vi "UI exit.vi"(0 "ZenGage v3.0 UI in":T2, 1 "SM_Stop_Stop_UI":bool, 5 "Event Registration Refnum":refnum<event-registration>, 7 "User Events Cluster_UI":T1, 9 "This VI":refnum<vi>, 11 "error in (no error)":errorcluster, 12 "SlaveLoop_UI":refnum<user-event>) -> (4 "ZenGage v3.0 UI out":T2, 6 "Stop Actor Loop":bool, 15 "error out":errorcluster)   [LabVIEW 2019, in "ZenGage v3.0 UI.lvclass"]
uses:
  ZenGage v3.0 UI.lvclass
  Type Definitions/User Events UI/Stop slave cluster.ctl
  Type Definitions/General/UI States(UI button enable disable).ctl
  Type Definitions/User Events UI/Optics diagnostics cluster.ctl
  <vilib>/vision/Image Controls.llb/IMAQ Image.ctl
  Type Definitions/User Events UI/LoadingBar_General_UI.ctl
  Type Definitions/User Events UI/UserEvents_UI.ctl
  Type Definitions/JSON Read/Data initialization.ctl
  Type Definitions/JSON Read/Post select init.ctl
  Type Definitions/Diagnostics/Trigger sensor.ctl
  Common/Controls/Pop-up Input.ctl
  Type Definitions/Inspection/Result Cluster.ctl
  Type Definitions/JSON Read/UI JSON read cluster.ctl
  Type Definitions/General/JSONRead.ctl
  Type Definitions/Inspection/Inspection Cluster.ctl
  Type Definitions/Diagnostics/Diagnostics(Cluster).ctl
  Type Definitions/Edit tolerance settings/Rack Selection.ctl
  <vilib>/Utility/miscctls.llb/LVPoint32TypeDef.ctl
  Type Definitions/Edit tolerance settings/Edit Tolerance Input.ctl
  Type Definitions/Edit tolerance settings/Edit Tolerance Overall Cluster.ctl
  Type Definitions/Controls and Indicators/Select a part (combobox).ctl
  Type Definitions/Controls and Indicators/EDL control references.ctl
  Type Definitions/Controls and Indicators/Diagnostics control referencs.ctl
  Type Definitions/Controls and Indicators/Inspection control references.ctl
  Type Definitions/Controls and Indicators/General_Control references.ctl
  Type Definitions/Controls and Indicators/Controls and Indicators Cluster.ctl
  Type Definitions/General/UIDataCluster.ctl
  Type Definitions/General/Master sample references.ctl
panel:
  # "e"
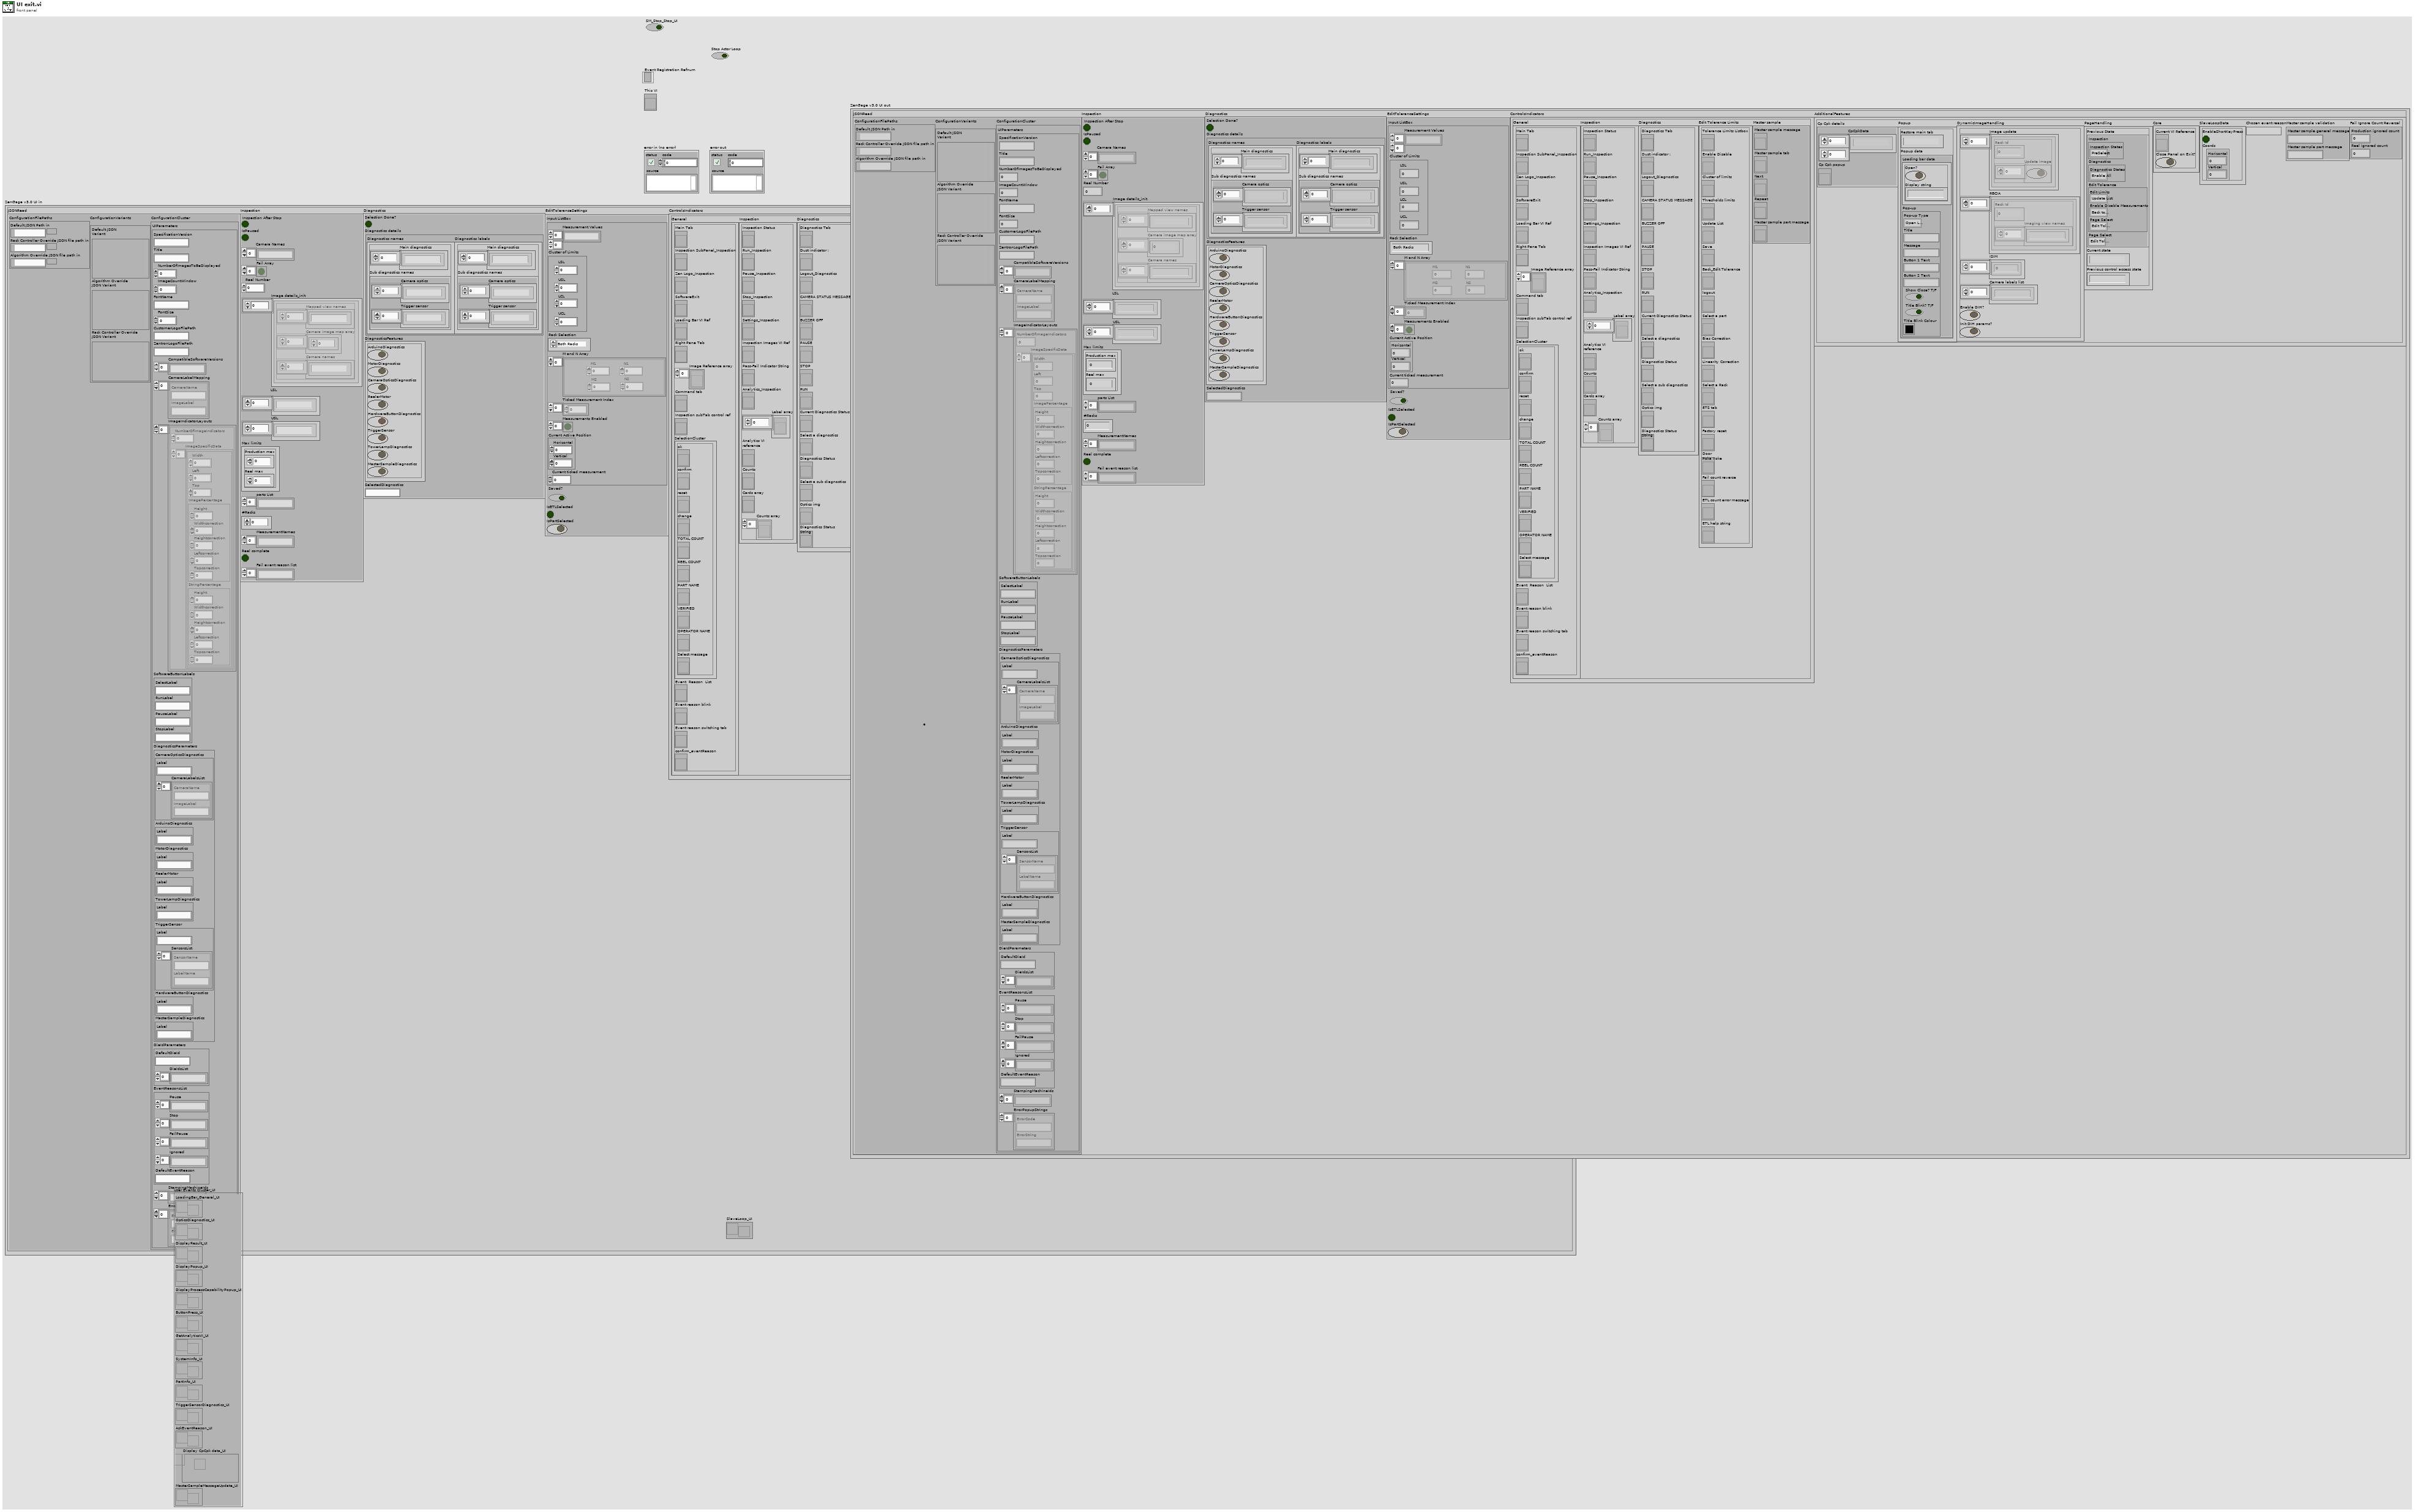
[diagram p1: front panel]
types:
  T1 = typedef "ZenGage v3.0 UI.lvclass/UserEvents_UI.ctl" = cluster{"LoadingBar_General_UI":refnum<user-event>, "OpticsDiagnostics_UI":refnum<user-event>, "DisplayResult_UI":refnum<user-event>, "DisplayPopup_UI":refnum<user-event>, "DisplayProcessCapabilityPopup_UI":refnum<user-event>, "ButtonPress_UI":refnum<user-event>, "GetAnalyticsVI_UI":refnum<user-event>, "SystemInfo_UI":refnum<user-event>, "PartInfo_UI":refnum<user-event>, "TriggerSensorDiagnostics_UI":refnum<user-event>, "AskEventReason_UI":refnum<user-event>, "Display CpCpk data_UI":refnum<user-event>, "MasterSampleMessageUpdate_UI":refnum<user-event>}
  T2 = typedef "UIDataCluster.ctl" = cluster{"JSONRead":T3, "Inspection":T5, "Diagnostics":T6, "EditToleranceSettings":T7, "ControlsIndicators":T11, "AdditionalFeatures":cluster{"Cp Cpk details":cluster{"CpCpkData":string[][], "Cp Cpk popup":refnum<vi>}, "Popup":cluster{"Restore main tab":string, "Popup data":cluster{"Loading bar data":cluster{"Open?":bool, "Display string":string}, "Pop-up":T17}}, "DynamicImageHandling":cluster{"Image update":cluster{"Rack Id":i32, "Update image":bool[]}[], "RBCIA":cluster{"Rack Id":u8, "Imaging view names":string[]}[], "ISIM":u8[], "Camera labels list":string[], "Enable DIH?":bool, "Init DIH params?":bool}, "PageHandling":cluster{"Previous State":T18, "Current state":string, "Previous control access state":string}, "Core":cluster{"Current VI Reference":refnum<vi>, "Close Panel on Exit?":bool}, "SlaveLoopData":cluster{"EnableShortKeyPress":bool, "Point32":T10}, "Chosen event reason":string, "Master sample validation":cluster{"Master sample general message":string, "Master sample part message":string}, "Fail Ignore Count Reversal":cluster{"Production ignored count":u64, "Reel ignored count":u64}}}
  T3 = typedef "ZenGage v3.0 UI.lvclass/JSONRead.ctl" = cluster{"ConfigurationFilePaths":cluster{"Default JSON Path in":path, "Rack Controller Override JSON file path in":path, "Algorithm Overrride JSON file path in ":path}, "ConfigurationVariants":cluster{"Default JSON \nVariant":variant, "Algorithm Override\nJSON Variant":variant, "Rack Controller Override\nJSON Variant":variant}, "ConfigurationCluster":T4}
  T4 = typedef "ZenGage v3.0 UI.lvclass/UI JSON read cluster.ctl" = cluster{"UIParameters":cluster{"SpecificationVersion":string, "Title":string, "NumberOfImagesToBeDisplayed":dbl, "ImageCountWindow":dbl, "FontName":string, "FontSize":dbl, "CustomerLogoFilePath":string, "ZentronLogoFilePath":string, "CompatibleSoftwareVersions":string[], "CameraLabelMapping":cluster{"CameraName":string, "ImageLabel":string}[], "ImageIndicatorLayouts":cluster{"NumberOfImageIndicators":dbl, "ImageSpecificData":cluster{"Width":dbl, "Left":dbl, "Top":dbl, "ImagePercentage":cluster{"Height":dbl, "Widthcorrection":i64, "Heightcorrection":i64, "Leftcorrection":dbl, "Topcorrection":dbl}, "StringPercentage":cluster{"Height":dbl, "Widthcorrection":i64, "Heightcorrection":dbl, "Leftcorrection":dbl, "Topcorrection":dbl}}[]}[], "SoftwareButtonLabels":cluster{"SelectLabel":string, "RunLabel":string, "PauseLabel":string, "StopLabel":string}, "DiagnosticsParameters":cluster{"CameraOpticsDiagnostics":cluster{"Label":string, "CameraLabelsList":cluster{"CameraName":string, "ImageLabel":string}[]}, "ArduinoDiagnostics":cluster{"Label":string}, "MotorDiagnostics":cluster{"Label":string}, "ReelerMotor":cluster{"Label":string}, "TowerLampDiagnostics":cluster{"Label":string}, "TriggerSensor":cluster{"Label":string, "SensorsList":cluster{"SensorName":string, "LabelName":string}[]}, "HardwareButtonDiagnostics":cluster{"Label":string}, "MasterSampleDiagnostics":cluster{"Label":string}}, "DieIdParameters":cluster{"DefaultDieId":string, "DieIdsList":string[]}, "EventReasonsList":cluster{"Pause":string[], "Stop":string[], "FailPause":string[], "Ignored":string[], "DefaultEventReason":string}, "StampingMachineIds":string[], "ErrorPopupStrings":cluster{"ErrorCode":string, "ErrorString":string}[]}}
  T5 = typedef "ZenGage v3.0 UI.lvclass/Inspection Cluster.ctl" = cluster{"Inspection After Stop":bool, "IsPaused":bool, "Camera Names":string[], "Fail Array":bool[], "Reel Number":u32, "Image details_init":cluster{"Mapped view names":string[], "Camera image map array":i32[], "Camera names":string[]}[], "LSL":string[], "USL":string[], "Max limits":cluster{"Production max":u64, "Reel max":u64}, "parts List":string[], "#Racks":u8, "MeasurementNames":string[], "Reel complete":bool, "Fail event reason list":string[]}
  T6 = typedef "ZenGage v3.0 UI.lvclass/Diagnostics(Cluster).ctl" = cluster{"Selection Done?":bool, "Diagnostics details":cluster{"Diagnostics names":cluster{"Main diagnostics":string[], "Sub diagnostics names":cluster{"Camera optics":string[], "Trigger sensor":string[]}}, "Diagnostics labels":cluster{"Main diagnostics":string[], "Sub diagnostics names":cluster{"Camera optics":string[], "Trigger sensor":string[]}}}, "DiagnosticsFeatures":cluster{"ArduinoDiagnostics":bool, "MotorDiagnostics":bool, "CameraOpticsDiagnostics":bool, "ReelerMotor":bool, "HardwareButtonDiagnostics":bool, "TriggerSensor":bool, "TowerLampDiagnostics":bool, "MasterSampleDiagnostics":bool}, "SelectedDiagnostics":string}
  T7 = typedef "ZenGage v3.0 UI.lvclass/Edit Tolerance Overall Cluster.ctl" = cluster{"Input ListBox":T8, "Saved?":bool, "IsETLSelected":bool, "IsPartSelected":bool}
  T8 = typedef "ZenGage v3.0 UI.lvclass/Edit Tolerance Input.ctl" = cluster{"Measurement Values":string[][], "Cluster of Limits":cluster{"LSL":dbl, "USL":dbl, "LCL":dbl, "UCL":dbl}, "Rack Selection":T9, "M and N Array":cluster{"M1":u64, "M2":u64, "N1":u64, "N2":u64}[], "Ticked Measurement Index":u32[], "Measurements Enabled":bool[], "Current Active Position":T10, "Current ticked measurement":dbl}
  T9 = typedef "ZenGage v3.0 UI.lvclass/Rack Selection.ctl" = enum16{"Both Racks", "Rack 2", "Rack 1"}
  T10 = typedef "LVPoint32TypeDef.ctl" = cluster{"Horizontal":i32, "Vertical":i32}
  T11 = typedef "ZenGage v3.0 UI.lvclass/Controls and Indicators Cluster.ctl" = cluster{"General":T12, "Inspection":T13, "Diagnostics":T14, "Edit Tolerance Limits":T15, "Master sample":T16}
  T12 = typedef "ZenGage v3.0 UI.lvclass/General_Control references.ctl" = cluster{"Main Tab":refnum<vi>, "Inspection SubPanel_Inspection":refnum<vi>, "Zen Logo_Inspection":refnum<vi>, "SoftwareExit":refnum<vi>, "Loading Bar VI Ref":refnum<vi>, "Right Pane Tab":refnum<vi>, "Image Reference array":refnum<vi>[], "Command tab":refnum<vi>, "Inspection subTab control ref":refnum<vi>, "SelectionCluster":cluster{"ok":refnum<vi>, "confirm":refnum<vi>, "reset":refnum<vi>, "change":refnum<vi>, "TOTAL COUNT":refnum<vi>, "REEL COUNT":refnum<vi>, "PART NAME":refnum<vi>, "VERIFIED":refnum<vi>, "OPERATOR NAME":refnum<vi>, "Select message":refnum<vi>}, "Event  Reason  List":refnum<vi>, "Event reason blink":refnum<vi>, "Event reason switching tab":refnum<vi>, "confirm_eventReason":refnum<vi>}
  T13 = typedef "ZenGage v3.0 UI.lvclass/Inspection control references.ctl" = cluster{"Inspection Status":refnum<vi>, "Run_Inspection":refnum<vi>, "Pause_Inspection":refnum<vi>, "Stop_Inspection":refnum<vi>, "Settings_Inspection":refnum<vi>, "Inspection Images VI Ref":refnum<vi>, "Pass-Fail Indicator String":refnum<vi>, "Analytics_Inspection":refnum<vi>, "Label array":refnum<vi>[], "Analytics VI\nreference":refnum<vi>, "Counts":refnum<vi>, "Cards array":refnum<vi>, "Counts array":refnum<vi>[]}
  T14 = typedef "ZenGage v3.0 UI.lvclass/Diagnostics control referencs.ctl" = cluster{"Diagnostics Tab":refnum<vi>, "Dust indicator :":refnum<vi>, "Logout_Diagnostics":refnum<vi>, "CAMERA STATUS MESSAGE":refnum<vi>, "BUZZER OFF":refnum<vi>, "PAUSE":refnum<vi>, "STOP":refnum<vi>, "RUN":refnum<vi>, "Current Diagnostics Status":refnum<vi>, "Select a diagnostics":refnum<vi>, "Diagnostics Status":refnum<vi>, "Select a sub diagnostics":refnum<vi>, "Optics img":refnum<vi>, "Diagnostics Status\nString":refnum<vi>}
  T15 = typedef "ZenGage v3.0 UI.lvclass/EDL control references.ctl" = cluster{"Tolerance Limits Listbox":refnum<vi>, "Enable Disable":refnum<vi>, "Cluster of limits":refnum<vi>, "Thresholds limits":refnum<vi>, "Update List":refnum<vi>, "Save":refnum<vi>, "Back_Edit Tolerance":refnum<vi>, "logout":refnum<vi>, "Select a part":refnum<vi>, "Bias Correction":refnum<vi>, "Linearity Correction":refnum<vi>, "Select a Rack":refnum<vi>, "ETS tab":refnum<vi>, "Factory reset":refnum<vi>, "Door\nPoka Yoke":refnum<vi>, "Fail count reverse":refnum<vi>, "ETL count error message":refnum<vi>, "ETL help string":refnum<vi>}
  T16 = typedef "Master sample references.ctl" = cluster{"Master sample message":refnum<vi>, "Master sample tab":refnum<vi>, "Next":refnum<vi>, "Repeat":refnum<vi>, "Master sample part message":refnum<vi>}
  T17 = typedef "Pop-up Input.ctl" = cluster{"Pop-up Type":enum16{"Open Logo Display", "Close Logo Display", "Open Loading Bar", "Close Loading Bar", "Open Alert Display", "Close Alert Display", "One button dialog box", "Two button dialog box", "User Authentication"}, "Title":string, "Message":string, "Button 1 Text":string, "Button 2 Text":string, "Show Close? T/F":bool, "Title Blink? T/F":bool, "Title Blink Colour":u32}
  T18 = typedef "ZenGage v3.0 UI.lvclass/UI States(UI button enable disable).ctl" = cluster{"Inspection":cluster{"Inspection States":enum16{"PreSelect", "Back _Inspection", "Analytics", "Ready To Run", "Ready To Insert", "Enable All buttons", "Disable All Buttons", "Settings", "Select", "Stop", "Pause", "Inspect"}}, "Diagnostics":cluster{"Diagnostics States":enum16{"Enable All", "Camera Optics Fail", "Loading Bar", "Camera Optics", "Motor", "Arduino", "POST Done", "POST"}}, "Edit Tolerance":cluster{"Edit Limits":enum16{"Update List"}, "Enable Disable Measurements":enum16{"Back to Edit Tolerance"}, "Page Select":enum16{"Edit Tolerance Limits", "Enable Disable Buttons"}}, "Page Select":enum16{"Edit Tolerance", "Diagnostics", "Inspection"}}
  T19 = typedef "ZenGage v3.0 UI.lvclass/Stop slave cluster.ctl" = cluster{"Stop UI?":bool}
  T20 = enum32{"Invalid", "Standard", "Closed", "Hidden", "Minimized", "Maximized"}
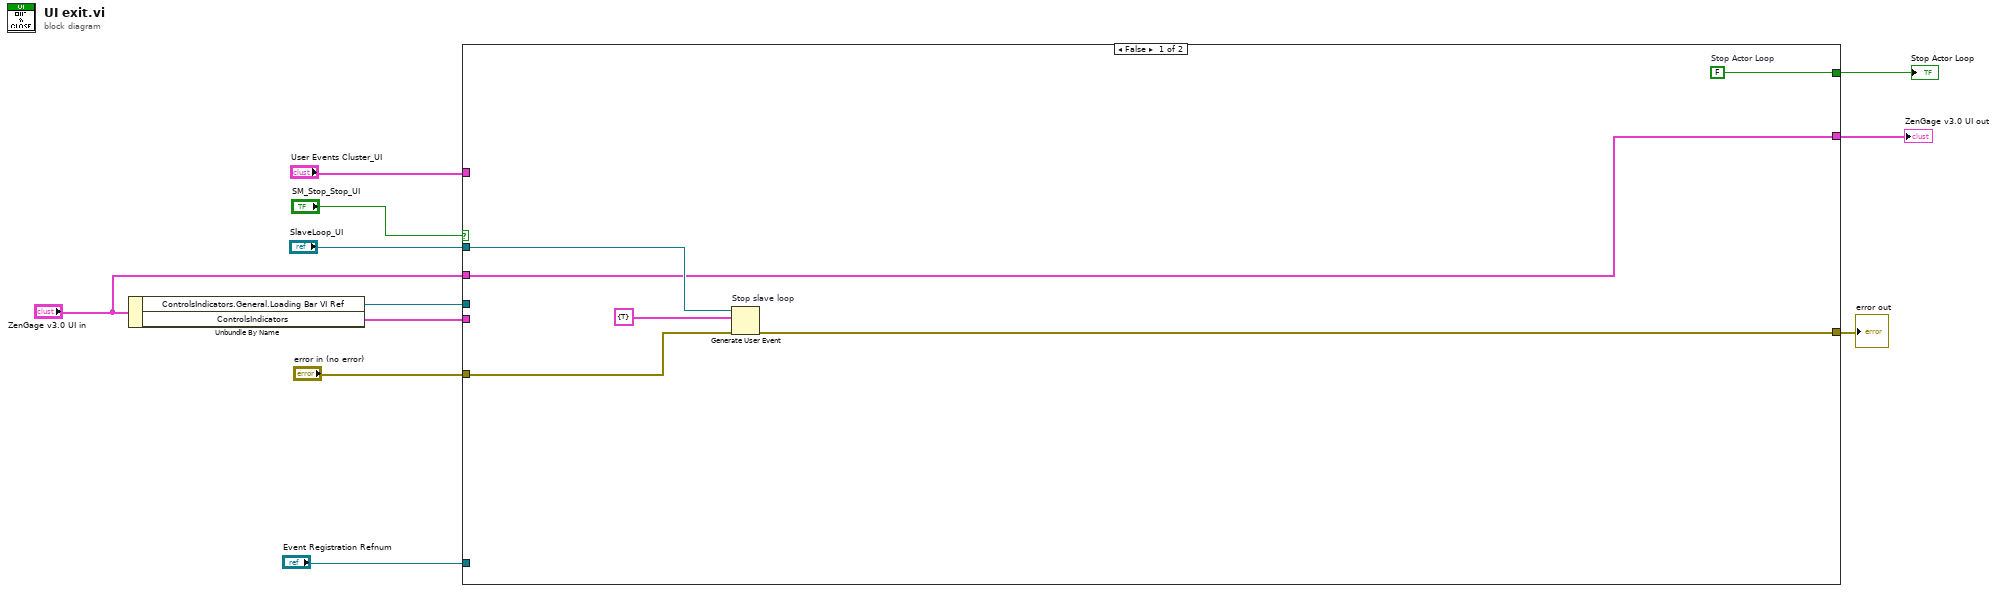
[diagram p0: block diagram]
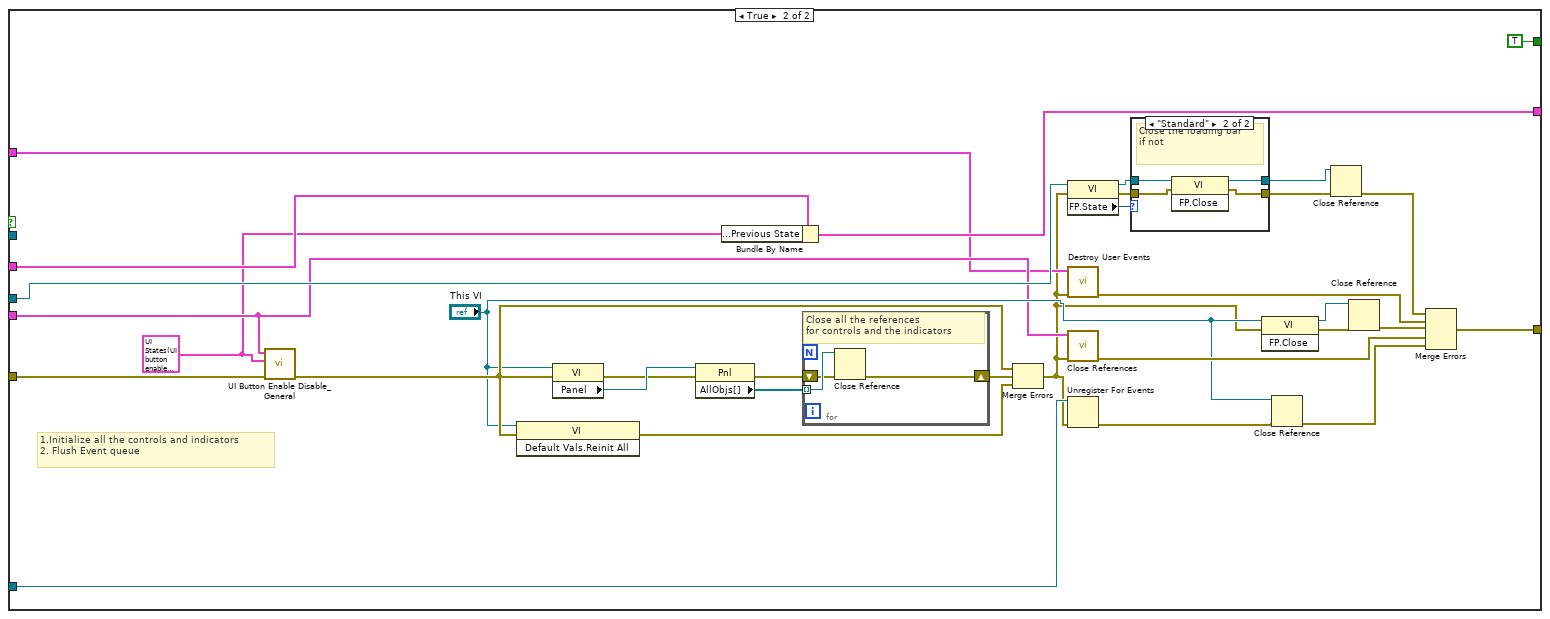
[diagram p2: hidden frame]
diagram:
  n1 = Unbundle By Name("ZenGage v3.0 UI in") -> ("ControlsIndicators.General.Loading Bar VI Ref"=w6:refnum<vi>, "ControlsIndicators"=w4:T11)
  n2 = case shown="False" "SM_Stop_Stop_UI" {
    tunnel: w6 -> [_ w49]
    tunnel: [w12 w25] -> w2
    tunnel: "error in (no error)" -> [w16 w42]
    tunnel: [w15 w18] -> w8
    tunnel: "Event Registration Refnum" -> [_ w34]
    tunnel: [w17 TRUE ("Stop Actor Loop")] -> w10
    tunnel: "SlaveLoop_UI" -> [w13 _]
    tunnel: w4 -> [_ w28]
    tunnel: "ZenGage v3.0 UI in" -> [w12 w27]
    tunnel: "User Events Cluster_UI" -> [_ w24]
    frame False {
      w17 = FALSE  # Stop Actor Loop
      n3 = Generate User Event "Stop slave loop"(user event=w13, event data cluster=T19 {"Stop UI?"=TRUE} ("event data"), error in=w16) -> (error out=w15:errorcluster)  [unwired: 1 in, 1 out]
    }
    frame True {
      w26 = T18 {"Inspection"={"Inspection States"=enum."Disable All Buttons"}, "Diagnostics"={"Diagnostics States"=enum."Enable All"}, "Edit Tolerance"={"Edit Limits"=enum."Update List", "Enable Disable Measurements"=enum."Back to Edit Tolerance", "Page Select"=enum."Edit Tolerance Limits"}, "Page Select"=enum."Inspection"} ("UI States")
      # "1.Initialize all the controls and indicators\n2. Flush Event queue"
      n4 = call "UI Button Enable Disable_General.vi"("Controls and Indicators\nReferences"=w28, "UI States"=w26, "error in (no error)"=w42) -> ("error out"=w31:errorcluster)  [unwired: 7 in]
      n5 = invoke class="VI" method="Default Vals.Reinit All"(reference="This VI", error in=w31) -> (error out=w35:errorcluster)  [unwired: 1 in, 2 out]
      n6 = property class="VI"(reference="This VI", error in=w31) -> (error out=w45:errorcluster, "Panel"=w47:refnum<vi>)  [unwired: 1 out]
      n7 = property class="Pnl"(reference=w47, error in=w45) -> (error out=w44:errorcluster, "AllObjs[]"=w46:refnum<vi>[])  [unwired: 1 out]
      n8 = Bundle By Name(cluster=w27, "AdditionalFeatures.PageHandling.Previous State"=w26) -> (w25:T2)
      n9 = for {
        tunnel: w46 -> [w52] mode=indexing
        shift-right: [w50] -> w40
        shift-left: w44 -> [w51]
        # "Close all the references\nfor controls and the indicators"
        n10 = Close Reference(reference=w52, error in (no error)=w51) -> (error out=w50:errorcluster)
      }
      n11 = Merge Errors(w31, w40, w35) -> (w21:errorcluster)
      n12 = property class="VI"(reference=w49, error in=w21) -> (reference out=w43:refnum<vi>, error out=w41:errorcluster, "FP.State"=w48:T20)
      n13 = call "Destroy User Events.vi"("error in (no error)"=w21, "User Events Cluster_UI"=w24) -> ("error out"=w33:errorcluster)  [unwired: 9 in]
      n14 = call "Close References.vi"("error in (no error)"=w21, "ZenGage v3.0 UI in"=w28) -> ("error out"=w36:errorcluster)  [unwired: 9 in]
      n15 = Unregister For Events(event registration refnum=w34, error in=w21) -> (error out=w20:errorcluster)
      n16 = case shown="\"Standard\"" w48 {
        tunnel: [w54 w57] -> w39
        tunnel: w43 -> [w53 w58]
        tunnel: w41 -> [w54 w56]
        tunnel: [w53 w55] -> w38
        frame "Invalid", Default {
        }
        frame "Standard" {
          # "Close the loading bar\nif not"
          n17 = invoke class="VI" method="FP.Close"(reference=w58, error in=w56) -> (reference out=w55:refnum<vi>, error out=w57:errorcluster)  [unwired: 1 in, 1 out]
        }
      }
      n18 = invoke class="VI" method="FP.Close"(reference="This VI", error in=w21) -> (reference out=w29:refnum<vi>, error out=w23:errorcluster)  [unwired: 1 in, 1 out]
      n19 = Close Reference(reference="This VI", error in (no error)=w20) -> (error out=w19:errorcluster)
      n20 = Close Reference(reference=w38, error in (no error)=w39) -> (error out=w37:errorcluster)
      n21 = Close Reference(reference=w29, error in (no error)=w23) -> (error out=w22:errorcluster)
      n22 = Merge Errors(w37, w33, w22, w36, w19) -> (w18:errorcluster)
    }
  }
  "Stop Actor Loop" <- w10
  "error out" <- w8
  "ZenGage v3.0 UI out" <- w2
